vi "PhotonPoseEstimator_EstimateAverageBestTargetsPose.vi"(10 "CameraResult":T15={"Targets"=[], "PhotonMultiTargetPNPResult"={"PhotonPNPResult"={"IsPresent"=FALSE, "bestReprojErr"=0.0, "altReprojErr"=0.0, "ambiguity"=0.0, "Best"={"TRANSLATION3D"={"X"=0.0, "Y"=0.0, "Z"=0.0}, "ROTATION3D"={"Q_quaternion"={"R"=1.0, "V"=[0.0, 0.0, 0.0]}}, "XF"=FALSE}, "Alt"={"TRANSLATION3D"={"X"=0.0, "Y"=0.0, "Z"=0.0}, "ROTATION3D"={"Q_quaternion"={"R"=1.0, "V"=[0.0, 0.0, 0.0]}}, "XF"=FALSE}}, "FiducialIDsUsed"=[]}, "PhotonPipelineMetadata"={"CaptureTimestampMicros"=0, "PublishTimestampMicros"=0, "SequenceID"=0, "TimeSinceLastPong"=0}} {"PhotonMultiTargetPNPResult"."PhotonPNPResult"."Alt"."TRANSLATION3D"."Z" format="%14.3f"; "PhotonMultiTargetPNPResult"."PhotonPNPResult"."Alt"."TRANSLATION3D"."Y" format="%14.3f"; "PhotonMultiTargetPNPResult"."PhotonPNPResult"."Alt"."TRANSLATION3D"."X" format="%14.3f"; "PhotonMultiTargetPNPResult"."PhotonPNPResult"."Best"."TRANSLATION3D"."Z" format="%14.3f"; "PhotonMultiTargetPNPResult"."PhotonPNPResult"."Best"."TRANSLATION3D"."Y" format="%14.3f"; "PhotonMultiTargetPNPResult"."PhotonPNPResult"."Best"."TRANSLATION3D"."X" format="%14.3f"; "Targets"."AltCameraToTarget"."TRANSLATION3D"."Z" format="%14.3f"; "Targets"."AltCameraToTarget"."TRANSLATION3D"."Y" format="%14.3f"; "Targets"."AltCameraToTarget"."TRANSLATION3D"."X" format="%14.3f"; "Targets"."BestCameraToTarget"."TRANSLATION3D"."Z" format="%14.3f"; "Targets"."BestCameraToTarget"."TRANSLATION3D"."Y" format="%14.3f"; "Targets"."BestCameraToTarget"."TRANSLATION3D"."X" format="%14.3f"}, 11 "PhotoPoseEstimator":T1={"LastPose"={"Translation3d"={"X"=0.0, "Y"=0.0, "Z"=0.0}, "Rotation3d"={"Q_quaternion"={"R"=1.0, "V"=[0.0, 0.0, 0.0]}}}, "ReferencePose"={"Translation3d"={"X"=0.0, "Y"=0.0, "Z"=0.0}, "Rotation3d"={"Q_quaternion"={"R"=1.0, "V"=[0.0, 0.0, 0.0]}}}, "FieldTags"={"AprilTagMap"={}, "FieldLength"=0.0, "FieldWidth"=0.0, "OriginPosition "=enum."kBlueAllianceWallRightSide,", "OriginPose3d"={"Translation3d"={"X"=0.0, "Y"=0.0, "Z"=0.0}, "Rotation3d"={"Q_quaternion"={"R"=1.0, "V"=[0.0, 0.0, 0.0]}}}}, "PrimaryStratety"=enum."LOWEST_AMBIGUITY", "Camera"="", "RobotToCamera"={"TRANSLATION3D"={"X"=0.0, "Y"=0.0, "Z"=0.0}, "ROTATION3D"={"Q_quaternion"={"R"=1.0, "V"=[0.0, 0.0, 0.0]}}, "XF"=FALSE}, "ReportedErrors"=[], "HighestAmbiguity"=10.0, "MultiTagFallbackStrategy"=enum."LOWEST_AMBIGUITY", "PoseCacheTimeoutSec"=-1.0, "PhotonTargetModel"={"Vertices"=[], "IsPlaner"=FALSE, "IsSpherical"=FALSE}, "BaseNTName"="/photonvision"} {"PhotonTargetModel"."Vertices"."Z" format="%14.3f"; "PhotonTargetModel"."Vertices"."Y" format="%14.3f"; "PhotonTargetModel"."Vertices"."X" format="%14.3f"; "RobotToCamera"."TRANSLATION3D"."Z" format="%14.3f"; "RobotToCamera"."TRANSLATION3D"."Y" format="%14.3f"; "RobotToCamera"."TRANSLATION3D"."X" format="%14.3f"; "FieldTags"."OriginPose3d"."Translation3d"."Z" format="%14.3f"; "FieldTags"."OriginPose3d"."Translation3d"."Y" format="%14.3f"; "FieldTags"."OriginPose3d"."Translation3d"."X" format="%14.3f"; "ReferencePose"."Translation3d"."Z" format="%14.3f"; "ReferencePose"."Translation3d"."Y" format="%14.3f"; "ReferencePose"."Translation3d"."X" format="%14.3f"; "LastPose"."Translation3d"."Z" format="%14.3f"; "LastPose"."Translation3d"."Y" format="%14.3f"; "LastPose"."Translation3d"."X" format="%14.3f"}) -> (1 "Pos Found":bool, 3 "PhotonEstimatedRobotPose":T12={"EstimatedPose"={"Translation3d"={"X"=0.0, "Y"=0.0, "Z"=0.0}, "Rotation3d"={"Q_quaternion"={"R"=1.0, "V"=[0.0, 0.0, 0.0]}}}, "TimeStamp_Seconds"=0.0, "targetsUsed"=[], "Strategy"=enum."LOWEST_AMBIGUITY"} {"targetsUsed"."AltCameraToTarget"."TRANSLATION3D"."Z" format="%14.3f"; "targetsUsed"."AltCameraToTarget"."TRANSLATION3D"."Y" format="%14.3f"; "targetsUsed"."AltCameraToTarget"."TRANSLATION3D"."X" format="%14.3f"; "targetsUsed"."BestCameraToTarget"."TRANSLATION3D"."Z" format="%14.3f"; "targetsUsed"."BestCameraToTarget"."TRANSLATION3D"."Y" format="%14.3f"; "targetsUsed"."BestCameraToTarget"."TRANSLATION3D"."X" format="%14.3f"; "EstimatedPose"."Translation3d"."Z" format="%14.3f"; "EstimatedPose"."Translation3d"."Y" format="%14.3f"; "EstimatedPose"."Translation3d"."X" format="%14.3f"})   [LabVIEW 2019, in "PhotonVisionLib.lvlib"]
doc: "This is an internal function. Use Update or Update_Pipeline instead of this function.\n\nDetermine the best target based the weighted average position of valid potential positions."
uses:
  PhotonVisionLib.lvlib
  <vilib>/Rock Robotics/WPI/ThirdParty/JAS_Junk/TrajLib/Trajectory_Library.lvlib
  <vilib>/Rock Robotics/WPI/ThirdParty/JAS_Junk/TrajLib/TypeDef/QUATERNION.ctl
  <vilib>/Rock Robotics/WPI/ThirdParty/JAS_Junk/TrajLib/TypeDef/ROTATION3D.ctl
  <vilib>/Rock Robotics/WPI/ThirdParty/JAS_Junk/TrajLib/TypeDef/TRANSLATION3D.ctl
  <vilib>/Rock Robotics/WPI/ThirdParty/JAS_Junk/TrajLib/TypeDef/POSE3D.ctl
  TypeDef/PhotonEstimatedRobotPoseType.ctl
  TypeDef/PhotonPoseEstimator_PotentialRobotLocation.ctl
  Enum/PhotonPoseStrategy_ENUM.ctl
  TypeDef/TargetCornerType.ctl
  <vilib>/Rock Robotics/WPI/ThirdParty/JAS_Junk/TrajLib/TypeDef/TRANSFORM3D.ctl
  TypeDef/PhotonTrackedTargetType.ctl
  TypeDef/PhotonPipelineResultType.ctl
  <vilib>/Rock Robotics/WPI/ThirdParty/JAS_Junk/TrajLib/TypeDef/AprilTag.ctl
  <vilib>/Rock Robotics/WPI/ThirdParty/JAS_Junk/TrajLib/Enum/AprilTagFieldLayoutOrignPosition_ENUM.ctl
  <vilib>/Rock Robotics/WPI/ThirdParty/JAS_Junk/TrajLib/TypeDef/AprilTagFieldLayout.ctl
  TypeDef/PhotonPoseEstimatorType.ctl
  TypeDef/PhotonPNPResultType.ctl
  TypeDef/PhotonMultiTargetPNPResultType.ctl
  TypeDef/PhotonTargetModel.ctl
  TypeDef/PhotonPipelineMetadataType.ctl
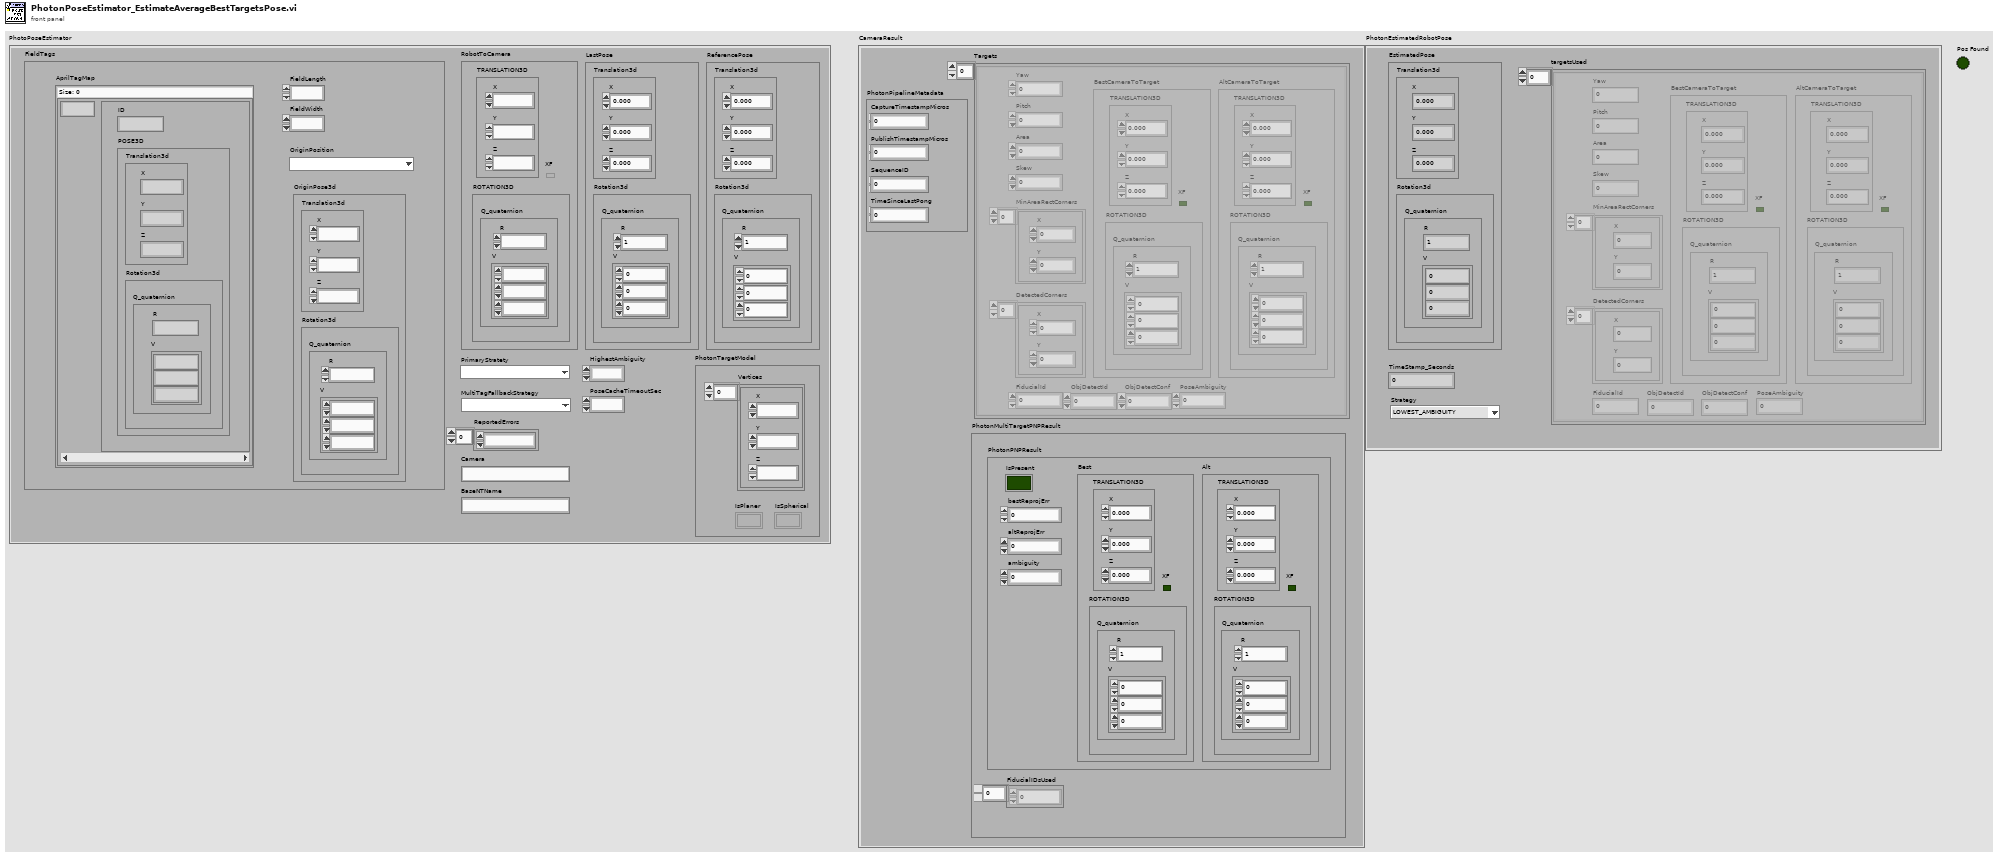
[diagram p1: front panel]
types:
  T1 = typedef "PhotonVisionLib.lvlib/PhotonPoseEstimatorType.ctl" = cluster{"LastPose":T2, "ReferencePose":T2, "FieldTags":T6, "PrimaryStratety":T9, "Camera":string, "RobotToCamera":T10, "ReportedErrors":dbl[], "HighestAmbiguity":dbl, "MultiTagFallbackStrategy":T9, "PoseCacheTimeoutSec":dbl, "PhotonTargetModel":T11, "BaseNTName":string}
  T2 = typedef "Trajectory_Library.lvlib/POSE3D.ctl" = cluster{"Translation3d":T3, "Rotation3d":T4}
  T3 = typedef "Trajectory_Library.lvlib/TRANSLATION3D.ctl" = cluster{"X":dbl, "Y":dbl, "Z":dbl}
  T4 = typedef "Trajectory_Library.lvlib/ROTATION3D.ctl" = cluster{"Q_quaternion":T5}
  T5 = typedef "Trajectory_Library.lvlib/QUATERNION.ctl" = cluster{"R":dbl, "V":dbl[]}
  T6 = typedef "Trajectory_Library.lvlib/AprilTagFieldLayout.ctl" = cluster{"AprilTagMap":map{i32, T7}, "FieldLength":dbl, "FieldWidth":dbl, "OriginPosition ":T8, "OriginPose3d":T2}
  T7 = typedef "Trajectory_Library.lvlib/AprilTag.ctl" = cluster{"ID":i32, "POSE3D":T2}
  T8 = typedef "Trajectory_Library.lvlib/AprilTagFieldLayoutOrignPosition_ENUM.ctl" = enum16{"kBlueAllianceWallRightSide,", "kRedAllianceWallRightSide,"}
  T9 = typedef "PhotonVisionLib.lvlib/PhotonPoseStrategy_ENUM.ctl" = enum16{"LOWEST_AMBIGUITY", "CLOSEST_TO_CAMERA_HEIGHT", "CLOSEST_TO_REFERENCE_POSE", "CLOSEST_TO_LAST_POSE", "AVERAGE_BEST_TARGETS", "MULTI_TAG_PNP_ON_COPROCESSOR", "MULTI_TAG_PNP_ON_RIO", "PNP_DISTANCE_TRIG_SOLVE", "CONSTRAINED_SOLVEPNP"}
  T10 = typedef "Trajectory_Library.lvlib/TRANSFORM3D.ctl" = cluster{"TRANSLATION3D":T3, "ROTATION3D":T4, "XF":bool}
  T11 = typedef "PhotonVisionLib.lvlib/PhotonTargetModel.ctl" = cluster{"Vertices":T3[], "IsPlaner":bool, "IsSpherical":bool}
  T12 = typedef "PhotonVisionLib.lvlib/PhotonEstimatedRobotPoseType.ctl" = cluster{"EstimatedPose":T2, "TimeStamp_Seconds":dbl, "targetsUsed":T13[], "Strategy":T9}
  T13 = typedef "PhotonVisionLib.lvlib/PhotonTrackedTargetType.ctl" = cluster{"Yaw":dbl, "Pitch":dbl, "Area":dbl, "Skew":dbl, "MinAreaRectCorners":T14[], "BestCameraToTarget":T10, "FiducialId":i32, "AltCameraToTarget":T10, "PoseAmbiguity":dbl, "DetectedCorners":T14[], "ObjDetectId":i32, "ObjDetectConf":sgl}
  T14 = typedef "PhotonVisionLib.lvlib/TargetCornerType.ctl" = cluster{"X":dbl, "Y":dbl}
  T15 = typedef "PhotonVisionLib.lvlib/PhotonPipelineResultType.ctl" = cluster{"Targets":T13[], "PhotonMultiTargetPNPResult":T16, "PhotonPipelineMetadata":T18}
  T16 = typedef "PhotonVisionLib.lvlib/PhotonMultiTargetPNPResultType.ctl" = cluster{"PhotonPNPResult":T17, "FiducialIDsUsed":i16[]}
  T17 = typedef "PhotonVisionLib.lvlib/PhotonPNPResultType.ctl" = cluster{"IsPresent":bool, "bestReprojErr":dbl, "altReprojErr":dbl, "ambiguity":dbl, "Best":T10, "Alt":T10}
  T18 = typedef "PhotonVisionLib.lvlib/PhotonPipelineMetadataType.ctl" = cluster{"CaptureTimestampMicros":i64, "PublishTimestampMicros":i64, "SequenceID":i64, "TimeSinceLastPong":i64}
  T19 = typedef "PhotonVisionLib.lvlib/PhotonPoseEstimator_PotentialRobotLocation.ctl" = cluster{"Inverse_Ambiguity":dbl, "PhotonEstimatedRobotPose":T12}
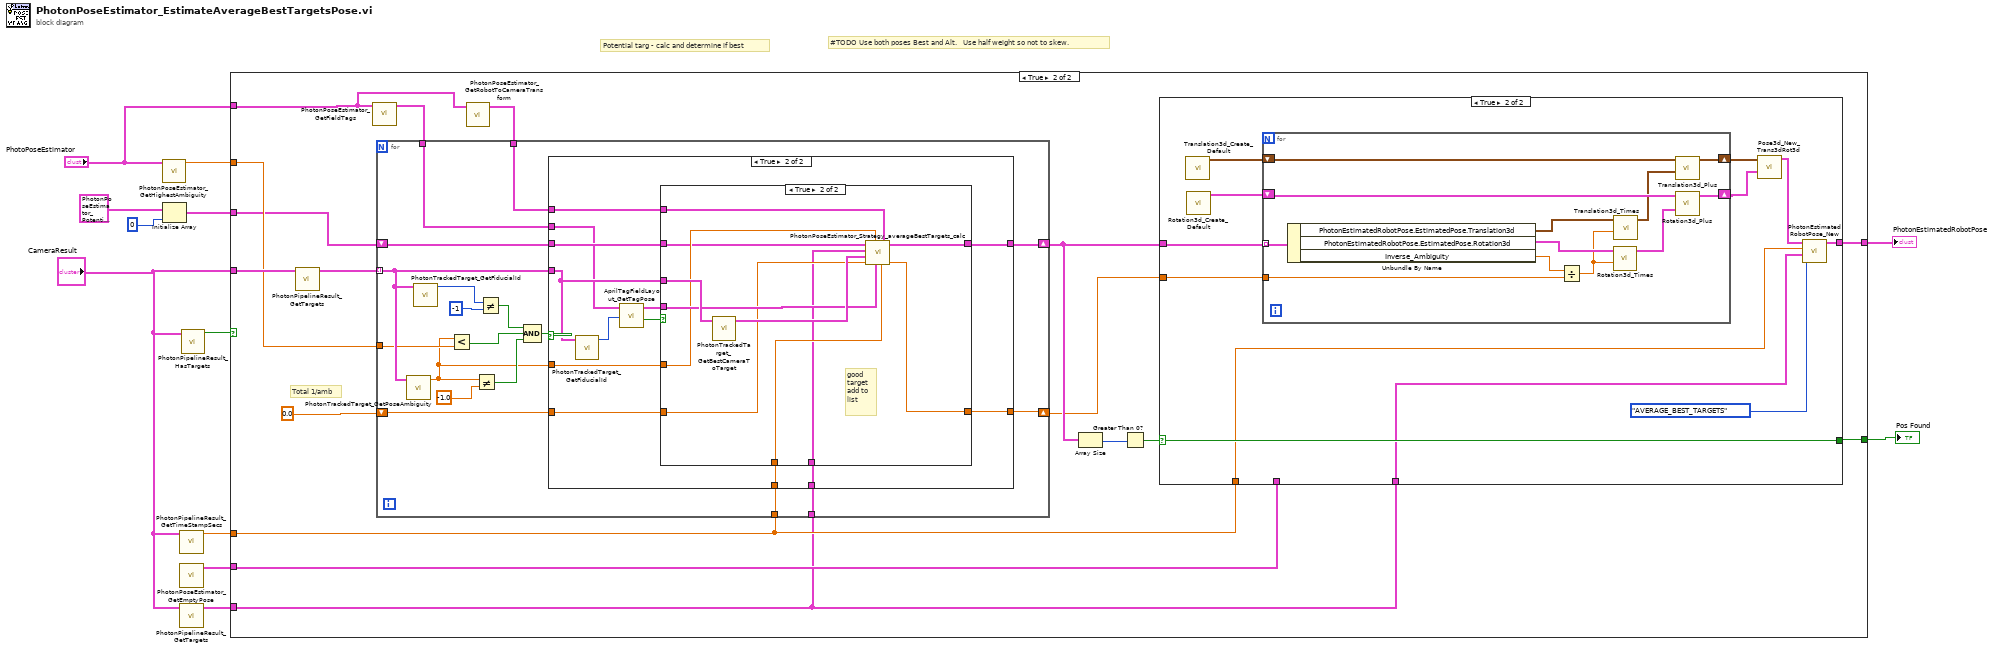
[diagram p0: block diagram]
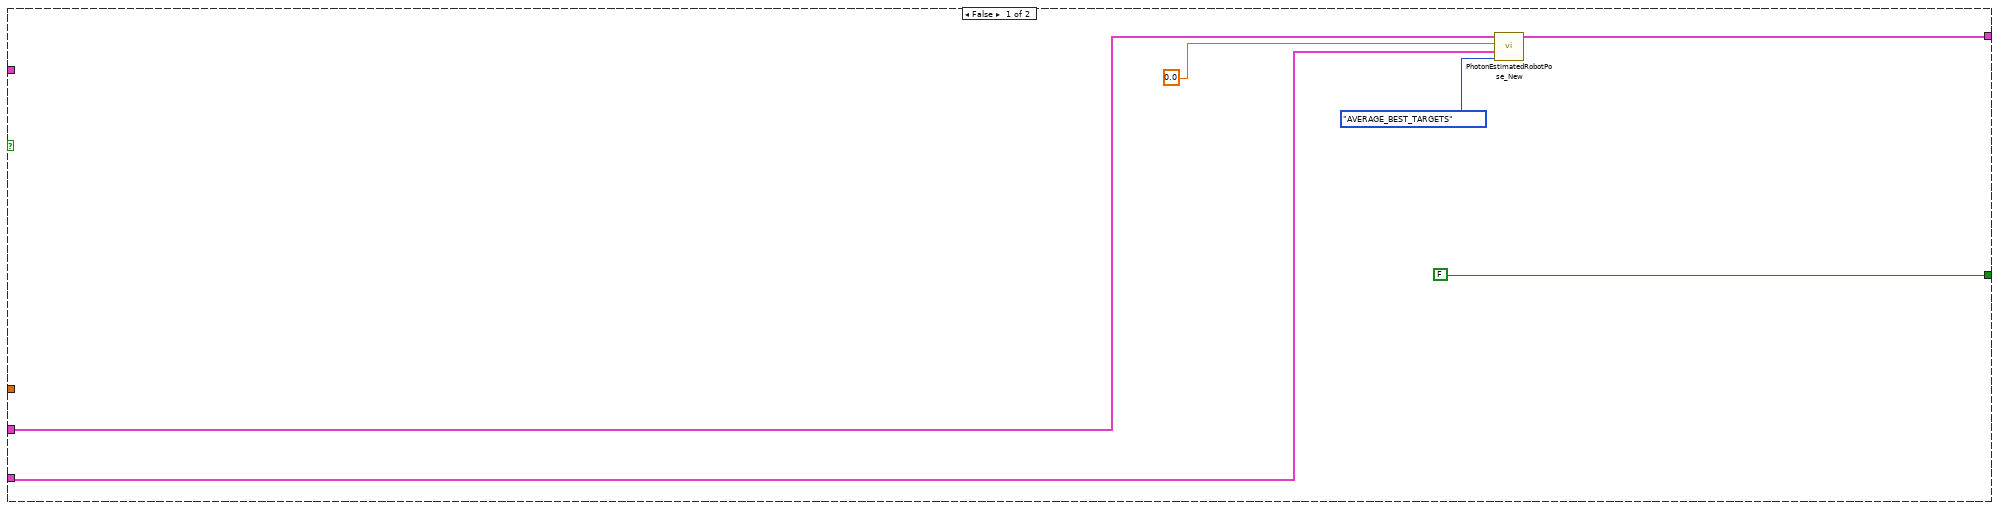
[diagram p2: hidden frame]
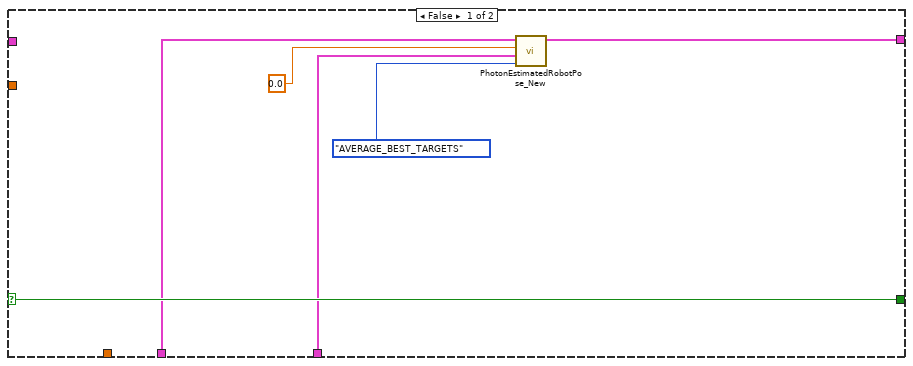
[diagram p3: hidden frame]
diagram:
  # "#TODO Use both poses Best and Alt.   Use half weight so not to skew."
  # "Potential targ - calc and determine if best"
  n1 = call "PhotonPoseEstimator_GetHighestAmbiguity.vi"("PhotonPoseEstimator"="PhotoPoseEstimator") -> ("HighestAmbiguity"=w9:dbl)  [unwired: 10 in]
  n2 = Initialize Array(T19 {"Inverse_Ambiguity"=0.0, "PhotonEstimatedRobotPose"={"EstimatedPose"={"Translation3d"={"X"=0.0, "Y"=0.0, "Z"=0.0}, "Rotation3d"={"Q_quaternion"={"R"=1.0, "V"=[0.0, 0.0, 0.0]}}}, "TimeStamp_Seconds"=0.0, "targetsUsed"=[], "Strategy"=enum."LOWEST_AMBIGUITY"}} ("PotentialRobotLocation"), 0 ("dimension size")) -> (w4:T19[])
  n3 = call "PhotonPipelineResult_GetTimeStampSecs.vi"("PhotonPipelineResult"="CameraResult") -> ("TimeStampSec"=w11:dbl)  [unwired: 10 in]
  n4 = call "PhotonPoseEstimator_GetEmptyPose.vi"() -> ("EmptyPose"=w10:T2)  [unwired: 11 in]
  n5 = call "PhotonPipelineResult_GetTargets.vi"("PhotonPipelineResult"="CameraResult") -> ("Targets"=w1:T13[])  [unwired: 10 in]
  n6 = call "PhotonPipelineResult_HasTargets.vi"("PhotonPipelineResult"="CameraResult") -> ("HasTargets"=w12:bool)  [unwired: 10 in]
  n7 = case shown="True" w12 {
    tunnel: "CameraResult" -> [_ w34]
    tunnel: [FALSE ("Found") w32] -> w7
    tunnel: "PhotoPoseEstimator" -> [_ w21]
    tunnel: w11 -> [_ w23]
    tunnel: w10 -> [w17 w31]
    tunnel: w9 -> [_ w30]
    tunnel: w4 -> [_ w29]
    tunnel: [w16 w25] -> w3
    tunnel: w1 -> [w13 w19]
    frame False {
      n8 = call "PhotonEstimatedRobotPose_New.vi"("Strategy"=PhotonPoseStrategy_ENUM."AVERAGE_BEST_TARGETS", "targetsUsed"=w13, "TimeStamp_Seconds"=0.0, "EstimatedPose"=w17) -> ("PhotonEstimatedRobotPose"=w16:T12)  [unwired: 7 in]
    }
    frame True {
      # "Total 1/amb"
      n9 = call "PhotonPipelineResult_GetTargets.vi"("PhotonPipelineResult"=w34) -> ("Targets"=w35:T13[])  [unwired: 10 in]
      n10 = call "PhotonPoseEstimator_GetFieldTags.vi"("PhotonPoseEstimator"=w21) -> ("AprilTagFieldLayout"=w22:T6)  [unwired: 10 in]
      n11 = call "PhotonPoseEstimator_GetRobotToCameraTransform.vi"("PhotonPoseEstimator"=w21) -> ("RobotToCamera"=w20:T10)  [unwired: 10 in]
      n12 = for {
        tunnel: w35 -> [w77] mode=indexing
        shift-right: [w81] -> w28
        shift-left: w29 -> [w80]
        shift-right: [w83] -> w24
        shift-left: 0.0 -> [w82]
        tunnel: w23 -> [w73]
        tunnel: w30 -> [w72]
        tunnel: w22 -> [w68]
        tunnel: w20 -> [w67]
        tunnel: w19 -> [w66]
        n13 = call "PhotonTrackedTarget_GetPoseAmbiguity.vi"("TrackedTarget"=w77) -> ("Pose Ambiguity"=w69:dbl)  [unwired: 10 in]
        n14 = call "PhotonTrackedTarget_GetFiducialId.vi"("TrackedTarget"=w77) -> ("Fiducial Id"=w79:i32)  [unwired: 10 in]
        n15 = Less?(x=w69, y=w72) -> (x < y?=w70:bool)
        n16 = Not Equal?(x=w69, y=-1.0) -> (x != y?=w75:bool)
        n17 = Not Equal?(x=w79, y=-1) -> (x != y?=w71:bool)
        n18 = Compound Arithmetic op=AND(w71, w70, w75) -> (w74:bool)
        n19 = case shown="True" w74 {
          tunnel: [w85 w97] -> w83
          tunnel: w82 -> [w85 w91]
          tunnel: w77 -> [_ w95]
          tunnel: [w84 w96] -> w81
          tunnel: w80 -> [w84 w98]
          tunnel: w73 -> [_ w90]
          tunnel: w69 -> [_ w89]
          tunnel: w68 -> [_ w88]
          tunnel: w67 -> [_ w87]
          tunnel: w66 -> [_ w86]
          frame False {
          }
          frame True {
            n20 = call "PhotonTrackedTarget_GetFiducialId.vi"("TrackedTarget"=w95) -> ("Fiducial Id"=w94:i32)  [unwired: 10 in]
            n21 = call <vilib>:"AprilTagFieldLayout_GetTagPose.vi"("TagId"=w94, "AprilTagFieldLayout"=w88) -> ("Found"=w93:bool, "TagPose3d"=w92:T2)  [unwired: 8 in]
            n22 = case shown="True" w93 {
              tunnel: w98 -> [w100 w104]
              tunnel: [w99 w103] -> w97
              tunnel: [w100 w110] -> w96
              tunnel: w95 -> [_ w109]
              tunnel: w92 -> [_ w108]
              tunnel: w91 -> [w99 w105]
              tunnel: w90 -> [_ w107]
              tunnel: w89 -> [_ w106]
              tunnel: w87 -> [_ w102]
              tunnel: w86 -> [_ w101]
              frame False {
              }
              frame True {
                # "good\ntarget\nadd to \nlist"
                n23 = call "PhotonTrackedTarget_GetBestCameraToTarget.vi"("TrackedTarget"=w109) -> ("BestCameraToTarget"=w111:T10)  [unwired: 9 in, 1 out]
                n24 = call "PhotonPoseEstimator_Strategy_averageBestTargets_calc.vi"("TimeStamp"=w107, "RobotToCamera"=w102, "FieldTargetPose"=w108, "Target Ambiguity"=w106, "In Total Inverse Amb"=w105, "TransformToEvaluate"=w111, "Targets"=w101, "In Potential Robot Loc"=w104) -> ("Out Total Inverse Amb"=w103:dbl, "Out Potential Robot Loc"=w110:T19[])  [unwired: 2 in]
              }
            }
          }
        }
      }
      n25 = Array Size(array=w28) -> (size(s)=w26:i32)
      n26 = Greater Than 0?(x=w26) -> (x > 0?=w27:bool)
      n27 = case shown="True" w27 {
        selector: w27 -> [w41 w53]
        tunnel: [w41 w53] -> w32
        tunnel: w28 -> [_ w52]
        tunnel: w31 -> [w39 _]
        tunnel: [w40 w46] -> w25
        tunnel: w24 -> [_ w51]
        tunnel: w23 -> [_ w44]
        tunnel: w19 -> [w37 w43]
        frame False {
          n28 = call "PhotonEstimatedRobotPose_New.vi"("Strategy"=PhotonPoseStrategy_ENUM."AVERAGE_BEST_TARGETS", "targetsUsed"=w37, "TimeStamp_Seconds"=0.0, "EstimatedPose"=w39) -> ("PhotonEstimatedRobotPose"=w40:T12)  [unwired: 7 in]
        }
        frame True {
          n29 = call <vilib>:"Translation3d_Create_Default.vi"() -> ("TRANSLATION3D"=w49:T3)  [unwired: 11 in]
          n30 = call <vilib>:"Rotation3d_Create_Default.vi"() -> ("ROTATION3D"=w50:T4)  [unwired: 11 in]
          n31 = for {
            tunnel: w52 -> [w65] mode=indexing
            tunnel: w51 -> [w63]
            shift-right: [w62] -> w47
            shift-left: w50 -> [w59]
            shift-right: [w61] -> w48
            shift-left: w49 -> [w60]
            n32 = Unbundle By Name(w65) -> ("PhotonEstimatedRobotPose.EstimatedPose.Translation3d"=w58:T3, "PhotonEstimatedRobotPose.EstimatedPose.Rotation3d"=w57:T4, "Inverse_Ambiguity"=w64:dbl)
            n33 = Divide(x=w64, y=w63) -> (x/y=w56:dbl)
            n34 = call <vilib>:"Rotation3d_Times.vi"("Scalar"=w56, "in Rotation3d"=w57) -> ("out Rotation3d"=w54:T4)  [unwired: 9 in]
            n35 = call <vilib>:"Translation3d_Times.vi"("Scalar"=w56, "In Translation3d"=w58) -> ("Out Translation3d"=w55:T3)  [unwired: 9 in]
            n36 = call <vilib>:"Translation3d_Plus.vi"("other Translation3d"=w55, "In Translation3d"=w60) -> ("Out Translation3d"=w61:T3)  [unwired: 9 in]
            n37 = call <vilib>:"Rotation3d_Plus.vi"("other Rotation3d"=w54, "in Rotation3d"=w59) -> ("out Rotation3d"=w62:T4)  [unwired: 9 in]
          }
          n38 = call <vilib>:"Pose3d_New_Trans3dRot3d.vi"("Rotation3d"=w47, "Translation3d"=w48) -> ("outPose3d"=w45:T2)  [unwired: 9 in]
          n39 = call "PhotonEstimatedRobotPose_New.vi"("Strategy"=PhotonPoseStrategy_ENUM."AVERAGE_BEST_TARGETS", "targetsUsed"=w43, "TimeStamp_Seconds"=w44, "EstimatedPose"=w45) -> ("PhotonEstimatedRobotPose"=w46:T12)  [unwired: 7 in]
        }
      }
    }
  }
  "PhotonEstimatedRobotPose" <- w3
  "Pos Found" <- w7
